vi "Handle Command.vi"(8 "error in (no error)":errorcluster, 9 "Data":variant, 10 "Command":string, 11 "Instrument.Example in":refnum<class "Instrument.Oxford1820.lvclass">) -> (0 "error out":errorcluster, 1 "Processed Data":variant, 2 "Command":string, 3 "Instrument.Example out":refnum<class "Instrument.Oxford1820.lvclass">)   [LabVIEW 2016, in "Instrument.Oxford1820.lvclass"]
uses:
  Instrument.Oxford1820.lvclass
  Instrument.Oxford1820.lvclass/Instrument.Oxford1820.ctl
  <userlib>/LevyLab/Levylab Instruments/Instrument Types/Cryostat/Instrument.Cryostat.lvclass
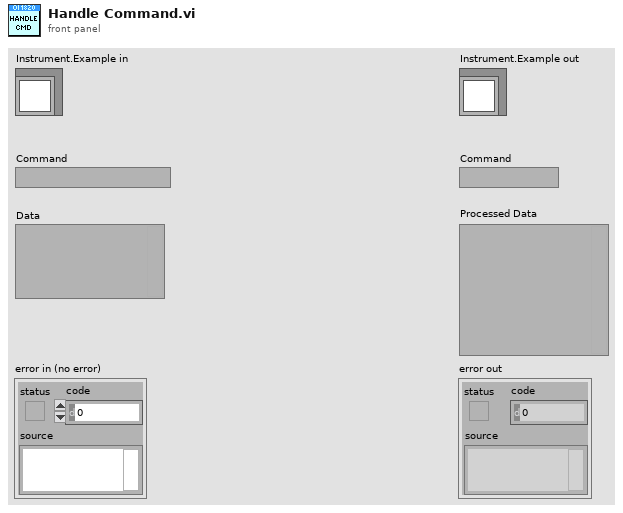
[diagram p1: front panel]
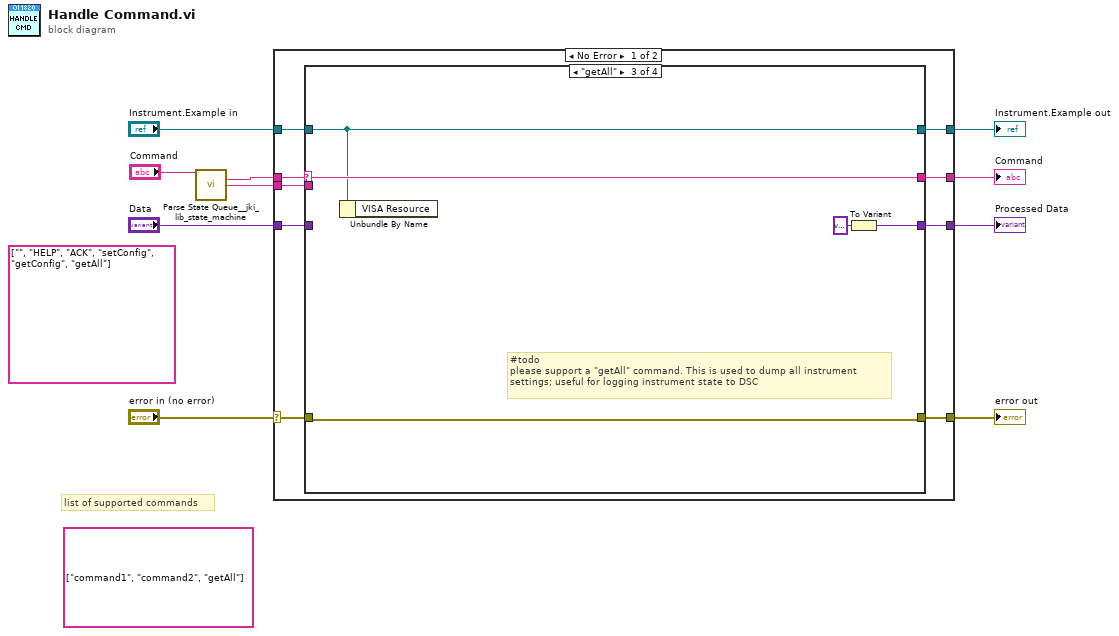
[diagram p0: block diagram]
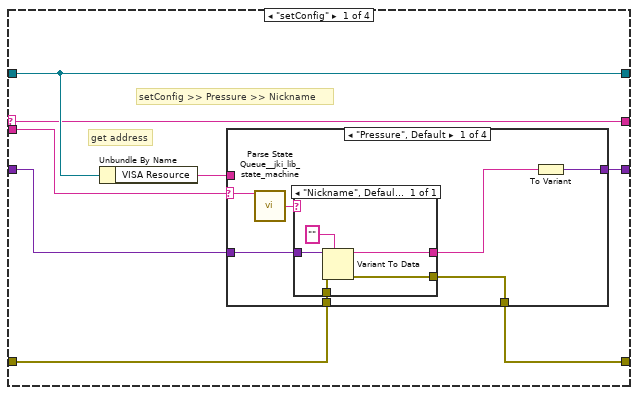
[diagram p2: hidden frame]
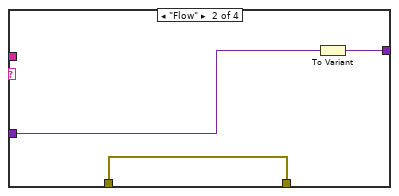
[diagram p3: hidden frame]
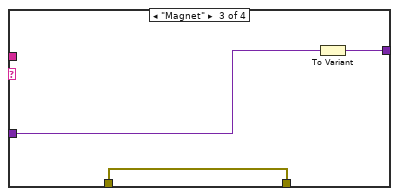
[diagram p4: hidden frame]
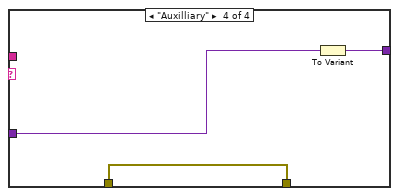
[diagram p5: hidden frame]
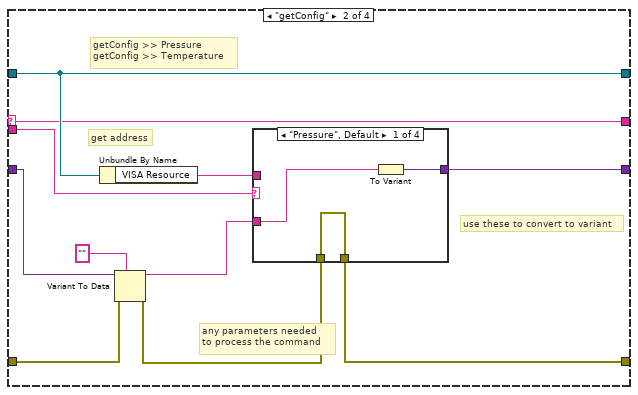
[diagram p6: hidden frame]
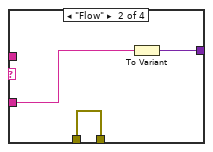
[diagram p7: hidden frame]
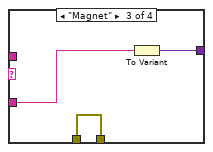
[diagram p8: hidden frame]
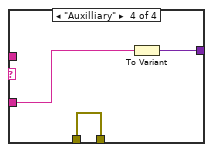
[diagram p9: hidden frame]
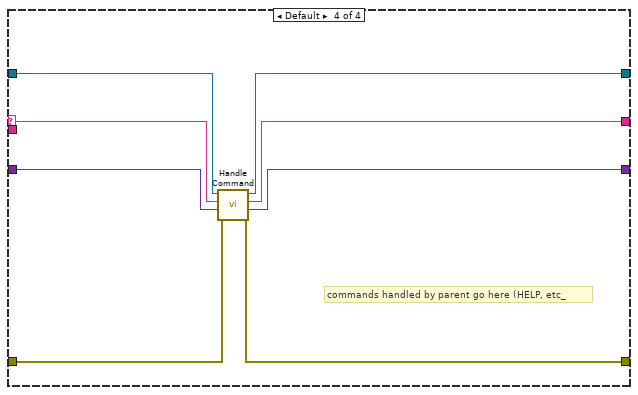
[diagram p10: hidden frame]
diagram:
  (unwired) string[] ["", "HELP", "ACK", "setConfig", "getConfig", "getAll"] ("Commands")
  (unwired) string[] ["command1", "command2", "getAll"] ("element")
  # "list of supported commands"
  n1 = call <vilib>:"Parse State Queue__jki_lib_state_machine.vi"("State Queue"="Command") -> ("Current State"=w2:string, "Arguments"=w1:string)  [unwired: 12 in, 1 out]
  n2 = case shown="No Error" "error in (no error)" {
    selector: "error in (no error)" -> [w14 w85]
    tunnel: [w13 w85] -> w10
    tunnel: [w19 _] -> w9
    tunnel: [w18 _] -> w8
    tunnel: [w17 w86] -> w7
    tunnel: "Data" -> [w16 _]
    tunnel: w2 -> [w12 _]
    tunnel: "Instrument.Example in" -> [w15 w86]
    tunnel: w1 -> [w11 _]
    frame No Error {
      n3 = case shown="\"getAll\"" w12 {
        selector: w12 -> [w25 w55 w76 w77]
        tunnel: [w26 w56 w75 w84] -> w19
        tunnel: [w25 w55 w76 w83] -> w18
        tunnel: [w27 w58 w73 w82] -> w17
        tunnel: w16 -> [w20 w59 _ w81]
        tunnel: w15 -> [w27 w58 w73 w80]
        tunnel: w14 -> [w21 w57 w74 w79]
        tunnel: [w24 w52 w74 w78] -> w13
        tunnel: w11 -> [w22 w50 _ _]
        frame "setConfig" {
          # "setConfig >> Pressure >> Nickname"
          # "get address"
          n4 = Unbundle By Name(w27) -> ("VISA Resource"=w23:string)
          n5 = case shown="\"Pressure\", Default" w22 {
            selector: w22 -> [w33 _ _ _]
            tunnel: [w34 w42 w45 w48] -> w26
            tunnel: [w29 w41 w44 w46] -> w24
            tunnel: w23 -> [_ _ _ _]
            tunnel: w21 -> [w31 w41 w44 w46]
            tunnel: w20 -> [w30 w40 w43 w47]
            frame "Pressure", Default {
              n6 = call <vilib>:"Parse State Queue__jki_lib_state_machine.vi"("State Queue"=w33) -> ("Arguments"=w32:string)  [unwired: 12 in, 2 out]
              n7 = case shown="\"Nickname\", Default" w32 {
                tunnel: w31 -> [w38]
                tunnel: [w37] -> w29
                tunnel: w30 -> [w36]
                tunnel: [w35] -> w28
                frame "Nickname", Default {
                  n8 = Variant To Data(error in=w38, type="" ("Command"), Variant=w36) -> (data=w35:string, error out=w37:errorcluster)
                }
              }
              n9 = To Variant(anything=w28) -> (Variant=w34:variant)
            }
            frame "Flow" {
              n10 = To Variant(anything=w40) -> (Variant=w42:variant)
            }
            frame "Magnet" {
              n11 = To Variant(anything=w43) -> (Variant=w45:variant)
            }
            frame "Auxilliary" {
              n12 = To Variant(anything=w47) -> (Variant=w48:variant)
            }
          }
        }
        frame "getConfig" {
          # "getConfig >> Pressure\ngetConfig >> Temperature"
          # "use these to convert to variant"
          # "any parameters needed\nto process the command"
          # "get address"
          n13 = Unbundle By Name(w58) -> ("VISA Resource"=w51:string)
          n14 = Variant To Data(error in=w57, type="" ("Command"), Variant=w59) -> (data=w49:string, error out=w53:errorcluster)
          n15 = case shown="\"Pressure\", Default" w50 {
            tunnel: [w62 w65 w68 w71] -> w56
            tunnel: w53 -> [w61 w63 w66 w69]
            tunnel: [w61 w63 w66 w69] -> w52
            tunnel: w51 -> [_ _ _ _]
            tunnel: w49 -> [w60 w64 w67 w70]
            frame "Pressure", Default {
              n16 = To Variant(anything=w60) -> (Variant=w62:variant)
            }
            frame "Flow" {
              n17 = To Variant(anything=w64) -> (Variant=w65:variant)
            }
            frame "Magnet" {
              n18 = To Variant(anything=w67) -> (Variant=w68:variant)
            }
            frame "Auxilliary" {
              n19 = To Variant(anything=w70) -> (Variant=w71:variant)
            }
          }
        }
        frame "getAll" {
          # "#todo\nplease support a \"getAll\" command. This is used to dump all instrument\nsettings; useful for logging instrument state to DSC"
          n20 = Unbundle By Name(w73) -> ()  [unwired: 1 out]
          n21 = To Variant(anything=variant ("variant")) -> (Variant=w75:variant)
        }
        frame Default {
          # "commands handled by parent go here (HELP, etc_"
          n22 = call-parent "Handle Command.vi"("error in (no error)"=w79, "Data"=w81, "Command"=w77, "Instrument in"=w80) -> ("error out"=w78:errorcluster, "Processed Data"=w84:variant, "Command"=w83:string, "Instrument out"=w82:refnum<class "Instrument.Oxford1820.lvclass">)  [unwired: 4 in]
        }
      }
    }
    frame Error {
    }
  }
  "error out" <- w10
  "Instrument.Example out" <- w7
  "Processed Data" <- w9
  "Command" <- w8
